vi "ips_readout.vi"() -> ()   [LabVIEW 2009]
panel:
  out "Measurement taken":bool
  in  "stop":bool
  out "Measured magnet current":string
  out "Measured Power supply":string
  out "Heartbeat":bool
  in  "stop 2":bool
  out "Current sweep rate":string
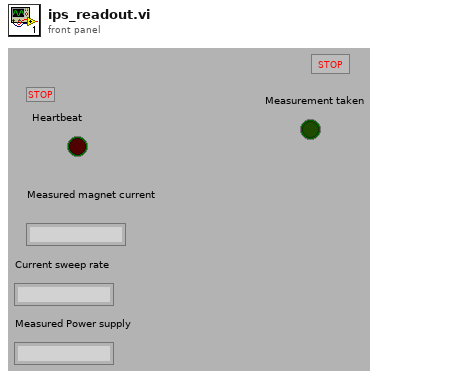
[diagram p1: front panel]
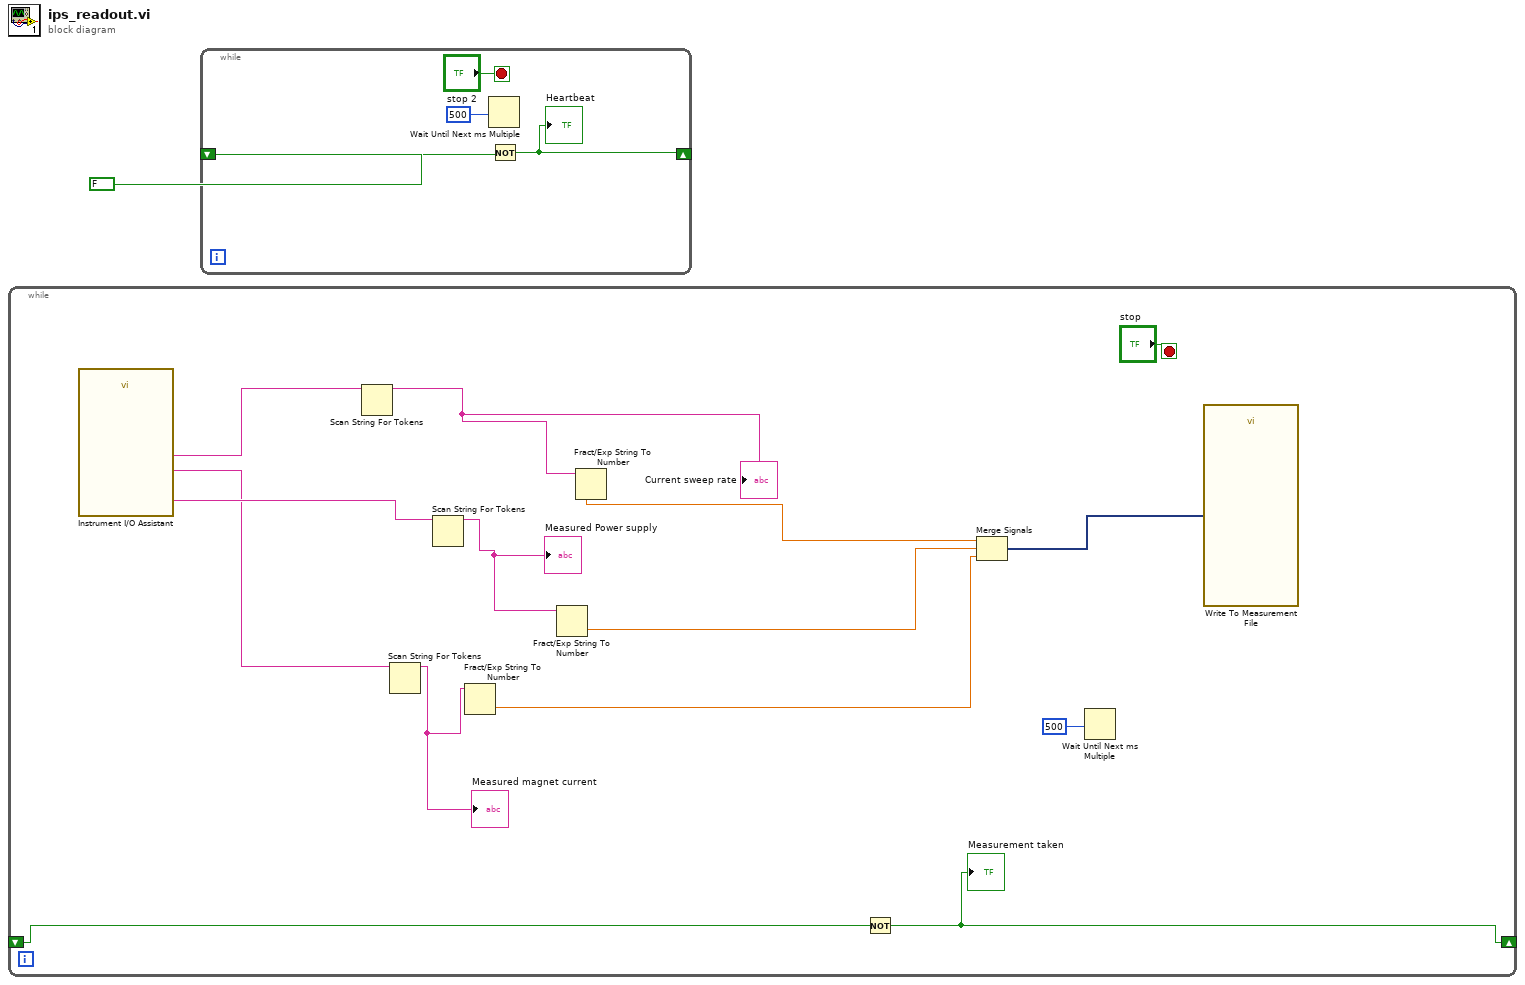
[diagram p0: block diagram]
diagram:
  n1 = while {
    shift-right: [w10] -> _
    shift-left: _ -> [w11]
    stop <- "stop" stop-if-true
    n2 = call "Instrument I/O Assistant"() -> ("Measured magnet current"=w12:string, "Current Sweep Rate"=w14:string, "Measured Measured Power Supply voltage"=w13:string)  [unwired: 23 in, 2 out]
    n3 = Scan String For Tokens(9:w14) -> (3:w7:string)  [unwired: 5 in, 3 out]
    "Current sweep rate" <- w7
    n4 = Scan String For Tokens(9:w12) -> (3:w3:string)  [unwired: 5 in, 3 out]
    "Measured magnet current" <- w3
    n5 = Scan String For Tokens(9:w13) -> (3:w5:string)  [unwired: 5 in, 3 out]
    "Measured Power supply" <- w5
    n6 = Fract/Exp String To Number(string=w3) -> (number=w2:dbl)  [unwired: 3 in, 1 out]
    n7 = Fract/Exp String To Number(string=w5) -> (number=w4:dbl)  [unwired: 3 in, 1 out]
    n8 = Fract/Exp String To Number(string=w7) -> (number=w6:dbl)  [unwired: 3 in, 1 out]
    n9 = Not(x=w11) -> (.not. x?=w10:bool)
    "Measurement taken" <- w10
    n10 = Merge Signals(w6, w4, w2) -> (w8:dynamicdata)
    n11 = Wait Until Next ms Multiple(millisecond multiple=500) -> ()  [unwired: 1 out]
    n12 = call "Write To Measurement File"("Signals"=w8) -> ()  [unwired: 16 in, 3 out]
  }
  n13 = while {
    shift-right: [w17] -> _
    shift-left: FALSE -> [w18]
    stop <- "stop 2" stop-if-true
    n14 = Wait Until Next ms Multiple(millisecond multiple=500) -> ()  [unwired: 1 out]
    n15 = Not(x=w18) -> (.not. x?=w17:bool)
    "Heartbeat" <- w17
  }
